vi "ELVIS III v1.0 AI Block Read Bank B.vi"(6 "CNT":u8, 7 "Bank Config":u8[](array[numeric]), 8 "error in (no error)":errorcluster, 9 "Count (tick/s)":u32, 10 "Number of Samples":u32=1000, 11 "AI Block Channels FPGA Reference":T1) -> (0 "error out":errorcluster, 3 "Data":dbl[][](array[numeric]))   [LabVIEW 2021]
uses:
  <vilib>/myRIO/Common/Instrument Driver Framework/ELVIS III v1.0/AI Block/typedefs/ELVIS III AI Block Channels FPGA Reference.ctl
  <vilib>/Utility/error.llb/Error Cluster From Error Code.vi
  <vilib>/rvi/errors/niLvFpgaAdjustHostInterfaceError.vi
  <vilib>/rvi/interface/nirviReadWriteControl/nirviReadWriteControl.xnode
  <vilib>/rvi/interface/nirviMethod/nirviMethod.xnode
  NiFpgaLv.dll
  <vilib>/rvi/interface/Simulation/niFpgaSimulationCallBeginRW.vi
  <vilib>/rvi/errors/niLvFpgaMergeErrorWithErrorCode.vi
  <vilib>/FPGAPlugInAG/Dynamic/niLvFpga_StartFifo_Dynamic.vi
  <vilib>/FPGAPlugInAG/Dynamic/niLvFpga_StopFifo_Dynamic.vi
  <vilib>/FPGAPlugInAG/Dynamic/niLvFpga_ReadFifo_Dynamic.vi
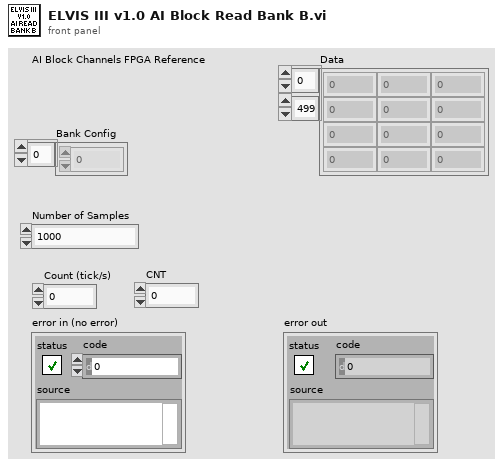
[diagram p1: front panel]
types:
  T1 = typedef "ELVIS III AI Block Channels FPGA Reference.ctl" = refnum<k20>
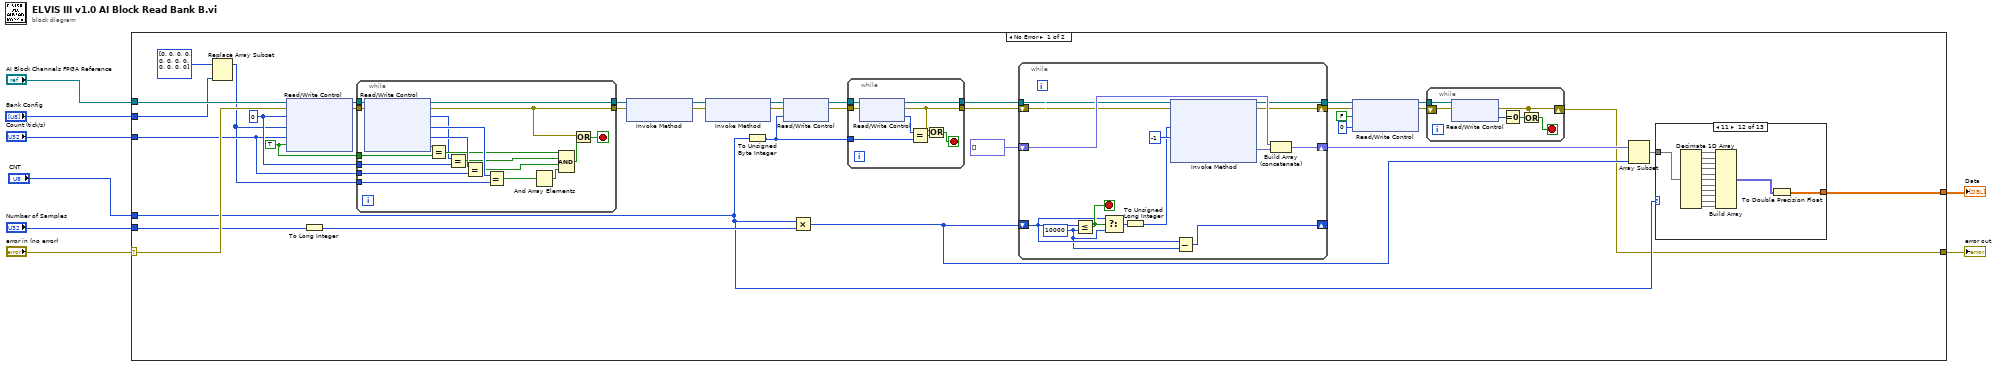
[diagram p0: block diagram]
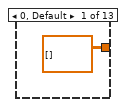
[diagram p2: hidden frame]
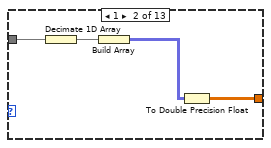
[diagram p3: hidden frame]
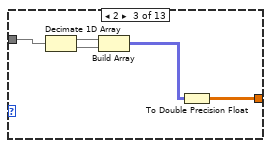
[diagram p4: hidden frame]
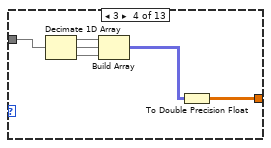
[diagram p5: hidden frame]
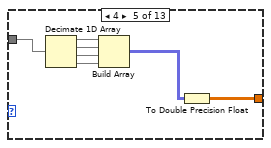
[diagram p6: hidden frame]
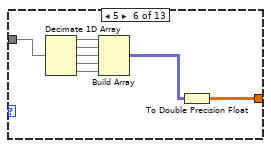
[diagram p7: hidden frame]
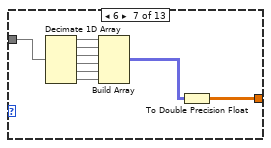
[diagram p8: hidden frame]
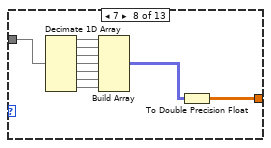
[diagram p9: hidden frame]
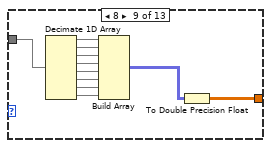
[diagram p10: hidden frame]
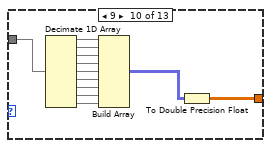
[diagram p11: hidden frame]
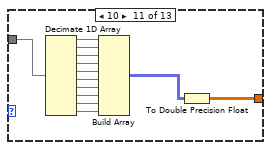
[diagram p12: hidden frame]
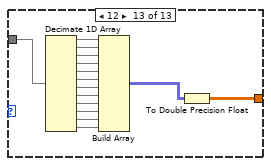
[diagram p13: hidden frame]
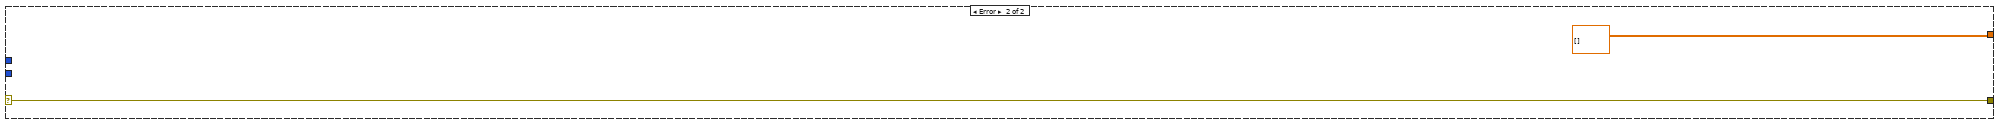
[diagram p14: hidden frame]
diagram:
  n1 = case shown="No Error" "error in (no error)" {
    selector: "error in (no error)" -> [w31 w207]
    tunnel: "AI Block Channels FPGA Reference" -> [w32 _]
    tunnel: "Count (tick/s)" -> [w22 _]
    tunnel: "Number of Samples" -> [w24 _]
    tunnel: "Bank Config" -> [w25 _]
    tunnel: [w37 dbl[][] [] ("Data")] -> w3
    tunnel: [w9 w207] -> w2
    tunnel: "CNT" -> [w13 _]
    frame No Error {
      w33 = TRUE ("AI.A.DMA_ENA")
      w27 = u8 0 ("AI.A.CNT")
      n2 = Replace Array Subset(array=u8[] [0, 0, 0, 0, 0, 0, 0, 0, 0, 0, 0, 0] ("AI.A.CNFG"), new element=w25) -> (w21:u8[])  [unwired: 1 in]
      n3 = xnode "Read/Write Control"("FPGA VI Reference In"=w32, "error in"=w31, "AI.B.CNT"=w27, "AI.B.CNFG"=w21, "AI.B.CNTR"=w22, "AI.B.DMA_ENA"=w33) -> ("FPGA VI Reference Out"=w34:T1, "error out"=w35:errorcluster)
      n4 = To Long Integer(number=w24) -> (32bit integer=w23:i32)
      n5 = while {
        tunnel: w34 -> [w83]
        tunnel: w35 -> [w82]
        tunnel: [w81] -> w30
        tunnel: [w73] -> w29
        tunnel: w21 -> [w71]
        tunnel: w22 -> [w79]
        tunnel: w27 -> [w77]
        tunnel: w33 -> [w68]
        stop <- w72 stop-if-true
        n6 = xnode "Read/Write Control"("FPGA VI Reference In"=w83, "error in"=w82) -> ("FPGA VI Reference Out"=w81:T1, "error out"=w73:errorcluster, "AI.B.CNT"=w66:u8, "AI.B.CNFG"=w80:u8[], "AI.B.CNTR"=w78:u32, "AI.B.DMA_ENA"=w69:bool)
        n7 = Equal?(x=w69, y=w68) -> (x = y?=w67:bool)
        n8 = Equal?(x=w66, y=w77) -> (x = y?=w76:bool)
        n9 = Equal?(x=w78, y=w79) -> (x = y?=w75:bool)
        n10 = Equal?(x=w80, y=w71) -> (x = y?=w65:bool[])
        n11 = And Array Elements(Boolean array=w65) -> (logical AND=w70:bool)
        n12 = Compound Arithmetic op=AND(w67, w76, w75, w70) -> (w74:bool)
        n13 = Or(x=w73, y=w74) -> (x .or. y?=w72:bool)
      }
      n14 = xnode "Invoke Method"("FPGA VI Reference In"=w30, "error in"=w29) -> ("FPGA VI Reference Out"=w44:T1, "error out"=w43:errorcluster)
      n15 = xnode "Invoke Method"("FPGA VI Reference In"=w44, "error in"=w43) -> ("FPGA VI Reference Out"=w42:T1, "error out"=w41:errorcluster)
      n16 = To Unsigned Byte Integer(number=w13) -> (unsigned 8bit integer=w36:u8)
      n17 = xnode "Read/Write Control"("FPGA VI Reference In"=w42, "error in"=w41, "AI.B.CNT"=w36) -> ("FPGA VI Reference Out"=w39:T1, "error out"=w40:errorcluster)
      n18 = Multiply(x=w13, y=w23) -> (x*y=w15:i32)
      n19 = while {
        tunnel: w40 -> [w206]
        tunnel: w39 -> [w205]
        tunnel: [w201] -> w19
        tunnel: [w204] -> w20
        tunnel: w36 -> [w202]
        stop <- w199 stop-if-true
        n20 = xnode "Read/Write Control"("FPGA VI Reference In"=w205, "error in"=w206) -> ("FPGA VI Reference Out"=w204:T1, "error out"=w201:errorcluster, "AI.B.CNT"=w203:u8)
        n21 = Equal?(x=w203, y=w202) -> (x = y?=w200:bool)
        n22 = Or(x=w201, y=w200) -> (x .or. y?=w199:bool)
      }
      n23 = while {
        tunnel: w20 -> [w54]
        shift-right: [w52] -> w17
        shift-left: w19 -> [w51]
        shift-right: [w57] -> w14
        shift-left: fxp<+/-,24,5>[] [] ("Data") -> [w58]
        shift-right: [w60] -> _
        shift-left: w15 -> [w62]
        tunnel: [w53] -> w18
        stop <- w63 stop-if-true
        w61 = 10000 ("y")
        n24 = Less Or Equal?(x=w62, y=w61) -> (x <= y?=w63:bool)
        n25 = Select(t=w62, s=w63, f=w61) -> (s? t:f=w56:i32)
        n26 = To Unsigned Long Integer(number=w56) -> (unsigned 32bit integer=w55:u32)
        n27 = xnode "Invoke Method"("FPGA VI Reference In"=w54, "error in"=w51, "Number of Elements"=w55, "Timeout (ms)"=-1) -> ("FPGA VI Reference Out"=w53:T1, "error out"=w52:errorcluster, "Data"=w59:fxp<+/-,24,5>[])  [unwired: 1 out]
        n28 = Subtract(x=w62, y=w61) -> (x-y=w60:i32)
        n29 = Build Array (concatenate)(w58, w59) -> (w57:fxp<+/-,24,5>[])
      }
      n30 = xnode "Read/Write Control"("FPGA VI Reference In"=w18, "error in"=w17, "AI.B.DMA_ENA"=FALSE ("Flag"), "AI.B.CNT"=u8 0) -> ("FPGA VI Reference Out"=w11:T1, "error out"=w10:errorcluster)
      n31 = while {
        tunnel: w11 -> [w50]
        shift-right: [w45] -> w9
        shift-left: w10 -> [w49]
        stop <- w46 stop-if-true
        n32 = xnode "Read/Write Control"("FPGA VI Reference In"=w50, "error in"=w49) -> ("error out"=w45:errorcluster, "AI.B.STAT"=w48:u8)  [unwired: 1 out]
        n33 = Equal To 0?(x=w48) -> (x = 0?=w47:bool)
        n34 = Or(x=w45, y=w47) -> (x .or. y?=w46:bool)
      }
      n35 = Array Subset(array=w14, length=w15) -> (w38:fxp<+/-,24,5>[])  [unwired: 1 in]
      n36 = case shown="11" w13 {
        tunnel: w38 -> [_ w88 w93 w99 w106 w114 w123 w133 w144 w156 w169 w183 w198]
        tunnel: [dbl[][] [] w86 w91 w97 w104 w112 w121 w131 w142 w154 w167 w181 w196] -> w37
        frame 0, Default {
        }
        frame 1 {
          n37 = Decimate 1D Array(w88) -> (w87:fxp<+/-,24,5>[])
          n38 = Build Array(w87) -> (w85:fxp<+/-,24,5>[][])
          n39 = To Double Precision Float(number=w85) -> (double precision float=w86:dbl[][])
        }
        frame 2 {
          n40 = Decimate 1D Array(w93) -> (w92:fxp<+/-,24,5>[], w89:fxp<+/-,24,5>[])
          n41 = Build Array(w92, w89) -> (w90:fxp<+/-,24,5>[][])
          n42 = To Double Precision Float(number=w90) -> (double precision float=w91:dbl[][])
        }
        frame 3 {
          n43 = Decimate 1D Array(w99) -> (w98:fxp<+/-,24,5>[], w95:fxp<+/-,24,5>[], w94:fxp<+/-,24,5>[])
          n44 = Build Array(w98, w95, w94) -> (w96:fxp<+/-,24,5>[][])
          n45 = To Double Precision Float(number=w96) -> (double precision float=w97:dbl[][])
        }
        frame 4 {
          n46 = Decimate 1D Array(w106) -> (w105:fxp<+/-,24,5>[], w102:fxp<+/-,24,5>[], w101:fxp<+/-,24,5>[], w100:fxp<+/-,24,5>[])
          n47 = Build Array(w105, w102, w101, w100) -> (w103:fxp<+/-,24,5>[][])
          n48 = To Double Precision Float(number=w103) -> (double precision float=w104:dbl[][])
        }
        frame 5 {
          n49 = Decimate 1D Array(w114) -> (w113:fxp<+/-,24,5>[], w110:fxp<+/-,24,5>[], w109:fxp<+/-,24,5>[], w108:fxp<+/-,24,5>[], w107:fxp<+/-,24,5>[])
          n50 = Build Array(w113, w110, w109, w108, w107) -> (w111:fxp<+/-,24,5>[][])
          n51 = To Double Precision Float(number=w111) -> (double precision float=w112:dbl[][])
        }
        frame 6 {
          n52 = Decimate 1D Array(w123) -> (w122:fxp<+/-,24,5>[], w119:fxp<+/-,24,5>[], w118:fxp<+/-,24,5>[], w117:fxp<+/-,24,5>[], w116:fxp<+/-,24,5>[], w115:fxp<+/-,24,5>[])
          n53 = Build Array(w122, w119, w118, w117, w116, w115) -> (w120:fxp<+/-,24,5>[][])
          n54 = To Double Precision Float(number=w120) -> (double precision float=w121:dbl[][])
        }
        frame 7 {
          n55 = Decimate 1D Array(w133) -> (w132:fxp<+/-,24,5>[], w129:fxp<+/-,24,5>[], w128:fxp<+/-,24,5>[], w127:fxp<+/-,24,5>[], w126:fxp<+/-,24,5>[], w125:fxp<+/-,24,5>[], w124:fxp<+/-,24,5>[])
          n56 = Build Array(w132, w129, w128, w127, w126, w125, w124) -> (w130:fxp<+/-,24,5>[][])
          n57 = To Double Precision Float(number=w130) -> (double precision float=w131:dbl[][])
        }
        frame 8 {
          n58 = Decimate 1D Array(w144) -> (w143:fxp<+/-,24,5>[], w140:fxp<+/-,24,5>[], w139:fxp<+/-,24,5>[], w138:fxp<+/-,24,5>[], w137:fxp<+/-,24,5>[], w136:fxp<+/-,24,5>[], w135:fxp<+/-,24,5>[], w134:fxp<+/-,24,5>[])
          n59 = Build Array(w143, w140, w139, w138, w137, w136, w135, w134) -> (w141:fxp<+/-,24,5>[][])
          n60 = To Double Precision Float(number=w141) -> (double precision float=w142:dbl[][])
        }
        frame 9 {
          n61 = Decimate 1D Array(w156) -> (w155:fxp<+/-,24,5>[], w152:fxp<+/-,24,5>[], w151:fxp<+/-,24,5>[], w150:fxp<+/-,24,5>[], w149:fxp<+/-,24,5>[], w148:fxp<+/-,24,5>[], w147:fxp<+/-,24,5>[], w146:fxp<+/-,24,5>[], w145:fxp<+/-,24,5>[])
          n62 = Build Array(w155, w152, w151, w150, w149, w148, w147, w146, w145) -> (w153:fxp<+/-,24,5>[][])
          n63 = To Double Precision Float(number=w153) -> (double precision float=w154:dbl[][])
        }
        frame 10 {
          n64 = Decimate 1D Array(w169) -> (w168:fxp<+/-,24,5>[], w165:fxp<+/-,24,5>[], w164:fxp<+/-,24,5>[], w163:fxp<+/-,24,5>[], w162:fxp<+/-,24,5>[], w161:fxp<+/-,24,5>[], w160:fxp<+/-,24,5>[], w159:fxp<+/-,24,5>[], w158:fxp<+/-,24,5>[], w157:fxp<+/-,24,5>[])
          n65 = Build Array(w168, w165, w164, w163, w162, w161, w160, w159, w158, w157) -> (w166:fxp<+/-,24,5>[][])
          n66 = To Double Precision Float(number=w166) -> (double precision float=w167:dbl[][])
        }
        frame 11 {
          n67 = Decimate 1D Array(w183) -> (w182:fxp<+/-,24,5>[], w179:fxp<+/-,24,5>[], w178:fxp<+/-,24,5>[], w177:fxp<+/-,24,5>[], w176:fxp<+/-,24,5>[], w175:fxp<+/-,24,5>[], w174:fxp<+/-,24,5>[], w173:fxp<+/-,24,5>[], w172:fxp<+/-,24,5>[], w171:fxp<+/-,24,5>[], w170:fxp<+/-,24,5>[])
          n68 = Build Array(w182, w179, w178, w177, w176, w175, w174, w173, w172, w171, w170) -> (w180:fxp<+/-,24,5>[][])
          n69 = To Double Precision Float(number=w180) -> (double precision float=w181:dbl[][])
        }
        frame 12 {
          n70 = Decimate 1D Array(w198) -> (w197:fxp<+/-,24,5>[], w194:fxp<+/-,24,5>[], w193:fxp<+/-,24,5>[], w192:fxp<+/-,24,5>[], w191:fxp<+/-,24,5>[], w190:fxp<+/-,24,5>[], w189:fxp<+/-,24,5>[], w188:fxp<+/-,24,5>[], w187:fxp<+/-,24,5>[], w186:fxp<+/-,24,5>[], w185:fxp<+/-,24,5>[], w184:fxp<+/-,24,5>[])
          n71 = Build Array(w197, w194, w193, w192, w191, w190, w189, w188, w187, w186, w185, w184) -> (w195:fxp<+/-,24,5>[][])
          n72 = To Double Precision Float(number=w195) -> (double precision float=w196:dbl[][])
        }
      }
    }
    frame Error {
    }
  }
  "error out" <- w2
  "Data" <- w3
